vi "main.vi"() -> ()   [LabVIEW 2024]
uses:
  controls/#typedef_octave.ctl
  controls/#typedef_program_data.ctl
  <vilib>/sound2/lvsound2.llb/Sound Output Task ID.ctl
  controls/#typedef_audio_settings.ctl
  <vilib>/sound2/lvsound2.llb/Sound Data Format.ctl
  controls/#typedef_monitoring.ctl
  controls/#typedef_wave_settings.ctl
  controls/#typedef_wave_types.ctl
  controls/#typedef_ProgramStates.ctl
  <vilib>/sound2/lvsound2.llb/Sampling Mode.ctl
  controls/#typedef_action_timer.ctl
  <vilib>/Analysis/3filter.llb/Filter Passband Type.ctl
  <extravilib>/ChannelInstances/Tag-bool/Write With Abort.vi
  <extravilib>/ChannelInstances/Tag-bool/Read With Abort.vi
  <extravilib>/ChannelInstances/Tag-bool/Instantiate.vi
  <vilib>/Utility/file.llb/Read Delimited Spreadsheet (DBL).vi
  <vilib>/Analysis/3filter.llb/Butterworth Filter (DBL).vi
  <vilib>/sound2/lvsound2.llb/Sound Output Write (DBL Single).vi
  <vilib>/Analysis/3filter.llb/Bessel Filter (DBL).vi
  <extravilib>/ChannelInstances/Tag-bool/EndpointRead.vi
  <extravilib>/ChannelInstances/Tag-bool/Endpoint.vi
  <vilib>/Utility/file.llb/Write Delimited Spreadsheet (DBL).vi
  <vilib>/Analysis/NI_AALPro.lvlib
  <extravilib>/ChannelInstances/Tag-bool.lvlib
  <vilib>/Analysis/NI_AALBase.lvlib
panel:
  out "error out 2":errorcluster
  in  "error in (no error) 2":errorcluster
  out "String":string
  out "NAME":string
  in  "Open":bool
  in  "Save":bool
  in  "ON/OFF":bool
  in  "Transpose  ch 2":i16(knob) caption="Octave" scale=-3.0..3.0
  in  "frequency ch2":i32(knob) caption="Transpose" scale=0.0..12.0
  in  "Wave type 2":u16(knob) caption="Wave type" scale=0.0..3.0
  in  "Blend":dbl(knob) scale=0.0..1.0
  in  "Transpose ch 1":i16(knob) caption="Octave" scale=-3.0..3.0
  in  "Wave type":u16(knob) scale=0.0..3.0
  in  "Distortion":dbl(knob)=1.0 scale=0.0..1.0
  in  "LOW freq":dbl(knob) scale=1.0..11024.0 scale format="%#_6p"
  in  "HI freq":dbl(knob)=11025.0 scale=1.0..11025.0 scale format="%#_6p"
  in  "Program Data":T1={"task ID"=0, "Data"=[], "Frequecies"=[], "Audio Settings"={"device ID"=0, "Buffer Size"=64.0, "sound format"={"sample rate (S/s)"=22050.0, "number of channels"=2, "bits per sample"=16}, "Number of samples"=0}, "Monitoring"={"Pressed Key Nr"=0, "Played Freqency"=0.0, "Max Amplitude"=0.0, "Current Amplitude"=0.0, "Played Freqency 2"=0.0, "Played Freqency drone"=0.0}, "Wave settings"={"HI freq"=0.0, "LOW freq"=0.0, "wave type"=enum."Sine", "Distortion level"=0.0, "MIX volume"=0.0, "wave type 2"=enum."Sine", "wave type drone"=enum."Sine", "DRONE volume 2"=0.0}, "data"=[]} {"task ID" format="%.0x"}
  out "Waveform Graph":waveform(dbl)(graph)
  in  "Volume":dbl(knob)=0.279 caption="Master volume" scale=0.0..1.0
  in  "Attack":dbl(knob)=5.930889758440234 scale=0.0..10.0
  in  "Decay":dbl(knob)=5.530816944711532 scale=0.0..10.0
  in  "Octave 2":T8
  in  "Octave":T8
  out "error out":errorcluster
  in  "error in (no error)":errorcluster
  # "Channel 1"
  # "Channel 2"
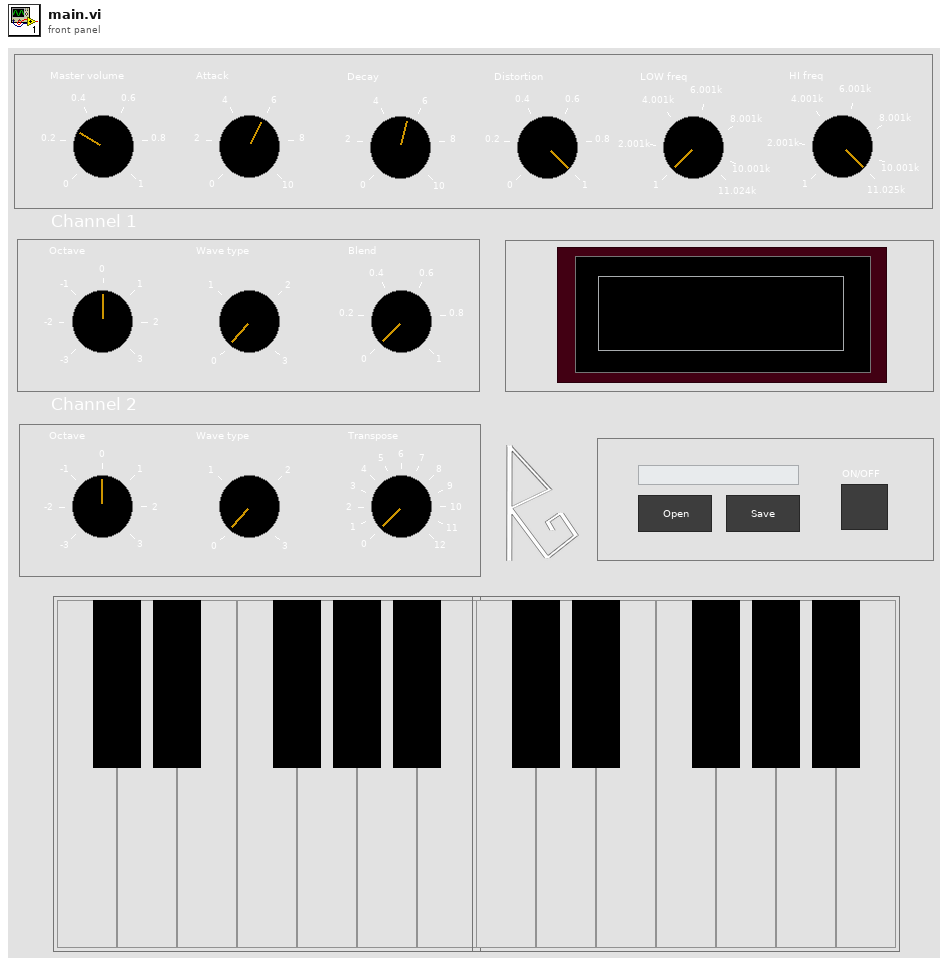
[diagram p1: front panel]
types:
  T1 = typedef "#typedef_program_data.ctl" = cluster{"task ID":T2, "Data":dbl[], "Frequecies":dbl[], "Audio Settings":T3, "Monitoring":T5, "Wave settings":T6, "data":waveform(dbl)[]}
  T2 = typedef "Sound Output Task ID.ctl" = u32
  T3 = typedef "#typedef_audio_settings.ctl" = cluster{"device ID":u32, "Buffer Size":dbl, "sound format":T4, "Number of samples":i32}
  T4 = typedef "Sound Data Format.ctl" = cluster{"sample rate (S/s)":dbl, "number of channels":i32, "bits per sample":i32}
  T5 = typedef "#typedef_monitoring.ctl" = cluster{"Pressed Key Nr":i32, "Played Freqency":dbl, "Max Amplitude":dbl, "Current Amplitude":dbl, "Played Freqency 2":dbl, "Played Freqency drone":dbl}
  T6 = typedef "#typedef_wave_settings.ctl" = cluster{"HI freq":dbl, "LOW freq":dbl, "wave type":T7, "Distortion level":dbl, "MIX volume":dbl, "wave type 2":T7, "wave type drone":T7, "DRONE volume 2":dbl}
  T7 = typedef "#typedef_wave_types.ctl" = enum16{"Sine", "Square", "Sawtooth", "Triangle"}
  T8 = typedef "#typedef_octave.ctl" = cluster{"C":bool, "D":bool, "E":bool, "F":bool, "G":bool, "C#":bool, "D#":bool, "A":bool, "G#":bool, "B":bool, "F#":bool, "Bb":bool}
  T9 = typedef "#typedef_ProgramStates.ctl" = enum16{"Application Error", "Settings", "Init", "logo", "Idle", "CheckNote", "Attack", "PlayNote", "Decay", "Release", "Exiting"}
  T10 = typedef "Tag-bool.lvlib/))Channel.ctl" = refnum<queue>
  T11 = typedef "#typedef_action_timer.ctl" = enum16{"reset", "timeElapsed"}
  T12 = typedef "NI_AALBase.lvlib/Filter Passband Type.ctl" = enum32{"Lowpass", "Highpass", "Bandpass", "Bandstop"}
  T13 = typedef "Sampling Mode.ctl" = i32
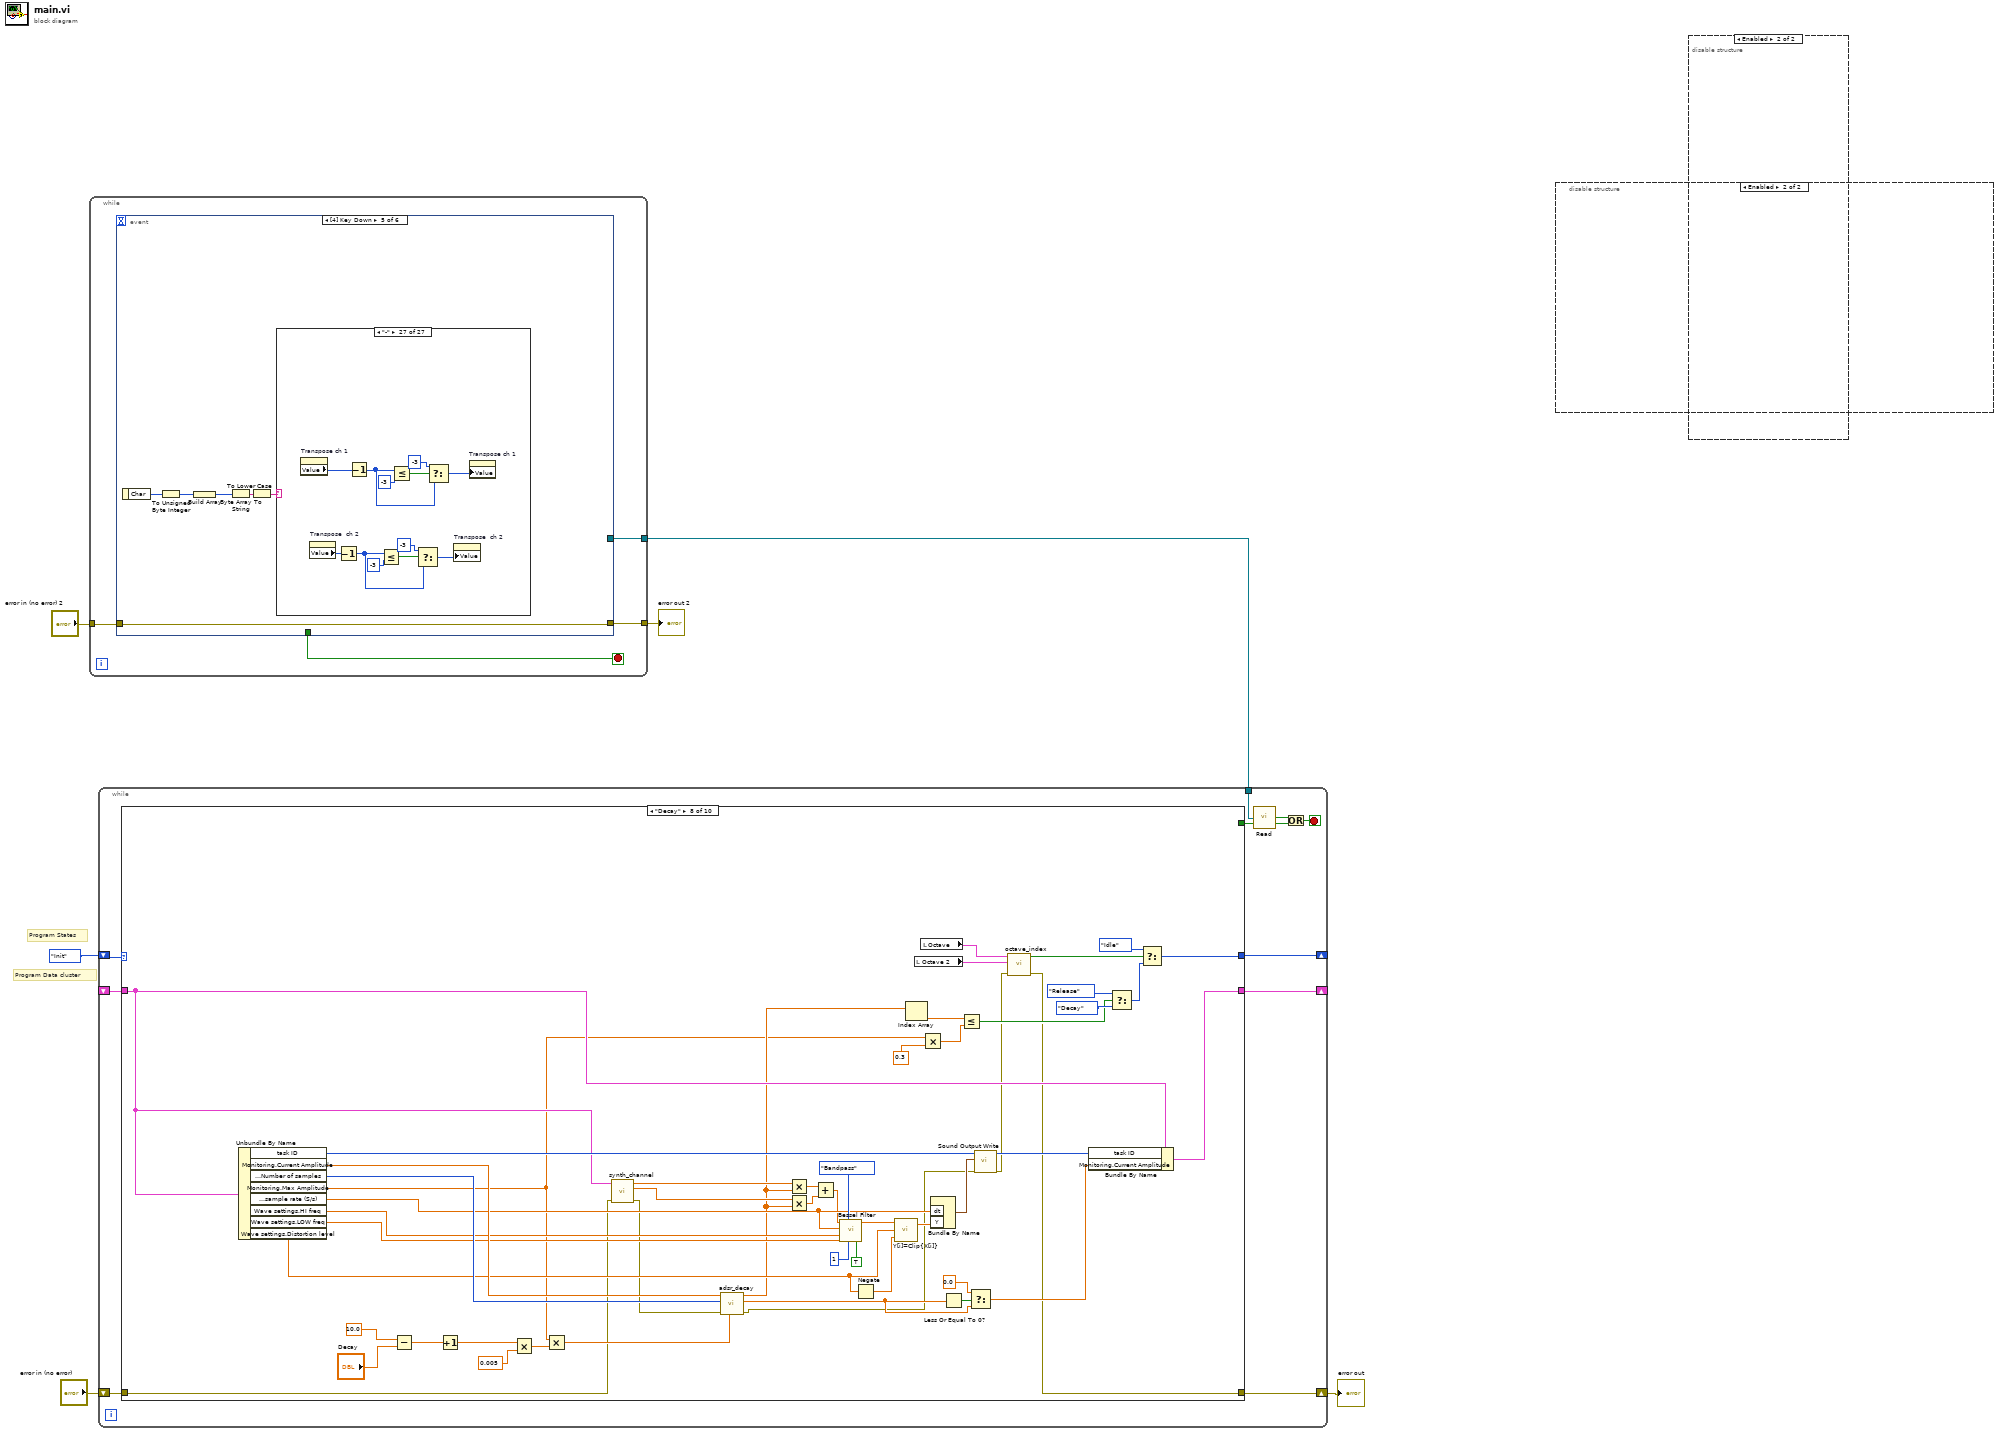
[diagram p0: block diagram]
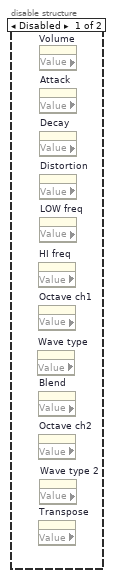
[diagram p2: hidden frame]
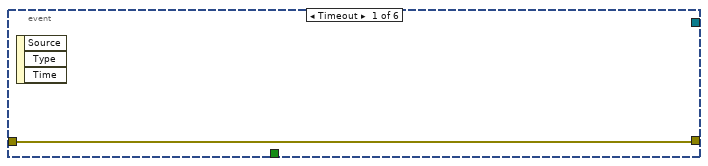
[diagram p3: hidden frame]
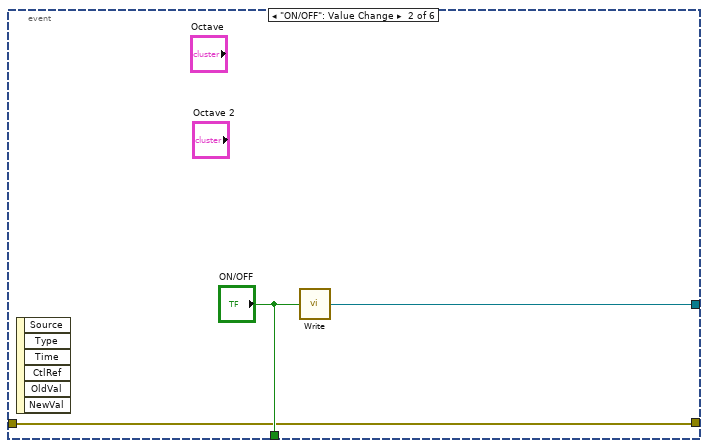
[diagram p4: hidden frame]
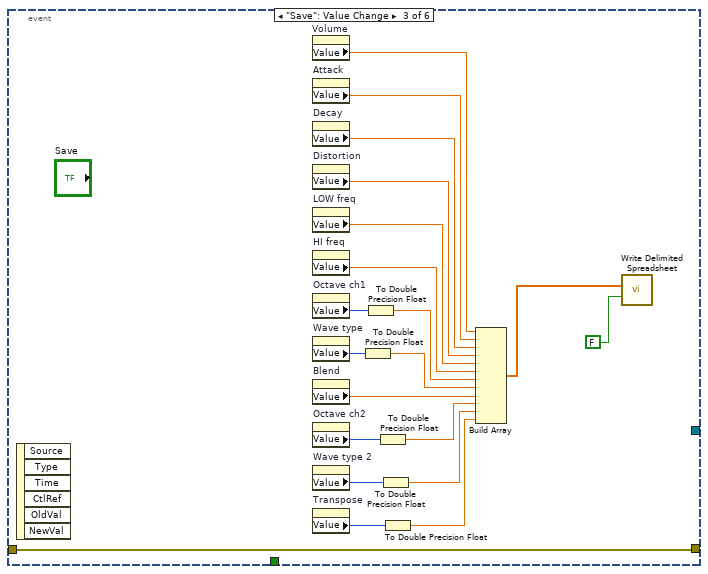
[diagram p5: hidden frame]
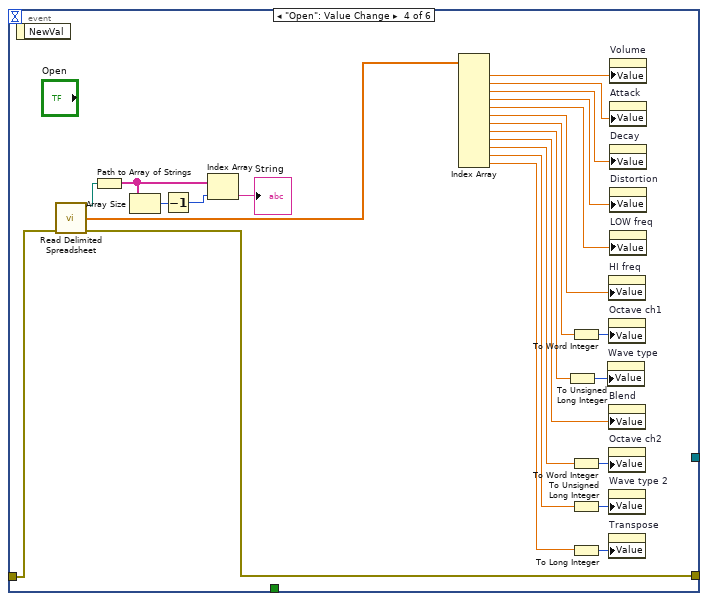
[diagram p6: hidden frame]
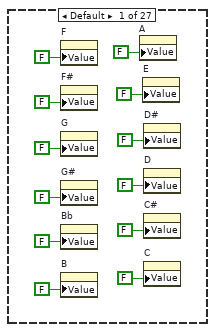
[diagram p7: hidden frame]
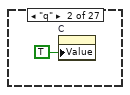
[diagram p8: hidden frame]
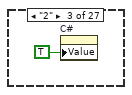
[diagram p9: hidden frame]
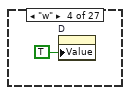
[diagram p10: hidden frame]
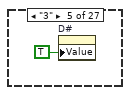
[diagram p11: hidden frame]
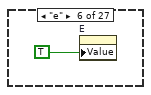
[diagram p12: hidden frame]
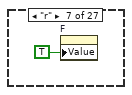
[diagram p13: hidden frame]
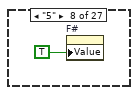
[diagram p14: hidden frame]
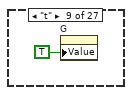
[diagram p15: hidden frame]
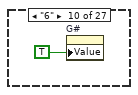
[diagram p16: hidden frame]
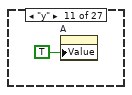
[diagram p17: hidden frame]
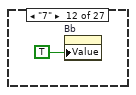
[diagram p18: hidden frame]
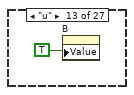
[diagram p19: hidden frame]
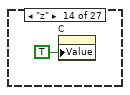
[diagram p20: hidden frame]
diagram:
  # "Program Data cluster"
  # "Program States"
  n1 = while {
    tunnel: [w9] -> w3
    tunnel: "error in (no error) 2" -> [w8]
    tunnel: [w7] -> w1
    stop <- w10 stop-if-true
    n2 = event shown="[4] Key Down" {
      selector: _ -> [_ _ _ _ _ _]
      dyn-events: _ -> [_ _ _ _ _ _]
      timeout: _ -> [_ _ _ _ _ _]
      tunnel: [_ "ON/OFF" _ _ _ _] -> w10
      tunnel: [_ w13 _ _ _ _] -> w9
      tunnel: w8 -> [w11 w12 w15 w54 w60 w126]
      tunnel: [w11 w12 w15 w53 w60 w126] -> w7
      event Timeout {
        n3 = event-data() -> ()  [unwired: 1 in, 3 out]
      }
      event "ON/OFF": Value Change {
        n4 = event-data() -> ()  [unwired: 1 in, 6 out]
        n5 = call <extravilib>:"Write.vi"("element"="ON/OFF") -> ("channel"=w13:T10)  [unwired: 1 out]
      }
      event "Save": Value Change {
        n6 = event-data() -> ()  [unwired: 1 in, 6 out]
        n7 = property on="Volume" class="Knob (strict)"() -> ("Value"=w32:dbl)  [unwired: 2 in, 2 out]
        n8 = property on="Attack" class="Knob (strict)"() -> ("Value"=w31:dbl)  [unwired: 2 in, 2 out]
        n9 = property on="Decay" class="Knob (strict)"() -> ("Value"=w30:dbl)  [unwired: 2 in, 2 out]
        n10 = property on="Distortion" class="Knob (strict)"() -> ("Value"=w29:dbl)  [unwired: 2 in, 2 out]
        n11 = property on="LOW freq" class="Knob (strict)"() -> ("Value"=w28:dbl)  [unwired: 2 in, 2 out]
        n12 = property on="HI freq" class="Knob (strict)"() -> ("Value"=w27:dbl)  [unwired: 2 in, 2 out]
        n13 = property on="Octave ch1" class="Knob (strict)"() -> ("Value"=w26:i16)  [unwired: 2 in, 2 out]
        n14 = property on="Wave type" class="Knob (strict)"() -> ("Value"=w17:u16)  [unwired: 2 in, 2 out]
        n15 = property on="Blend" class="Knob (strict)"() -> ("Value"=w25:dbl)  [unwired: 2 in, 2 out]
        n16 = property on="Octave ch2" class="Knob (strict)"() -> ("Value"=w24:i16)  [unwired: 2 in, 2 out]
        n17 = property on="Wave type 2" class="Knob (strict)"() -> ("Value"=w16:u16)  [unwired: 2 in, 2 out]
        n18 = property on="Transpose" class="Knob (strict)"() -> ("Value"=w23:i32)  [unwired: 2 in, 2 out]
        n19 = To Double Precision Float(number=w17) -> (double precision float=w19:dbl)
        n20 = To Double Precision Float(number=w26) -> (double precision float=w18:dbl)
        n21 = To Double Precision Float(number=w24) -> (double precision float=w20:dbl)
        n22 = To Double Precision Float(number=w16) -> (double precision float=w21:dbl)
        n23 = To Double Precision Float(number=w23) -> (double precision float=w22:dbl)
        n24 = Build Array(w32, w31, w30, w29, w28, w27, w18, w19, w25, w20, w21, w22) -> (w33:dbl[])
        n25 = call-poly <vilib>:"Write Delimited Spreadsheet.vi"("1D data"=w33, "append to file? (new file:F)"=FALSE) -> ()  [unwired: 12 in, 2 out]
      }
      event "Open": Value Change {
        n26 = event-data() -> ()  [unwired: 1 in, 1 out]
        n27 = call-poly <vilib>:"Read Delimited Spreadsheet.vi"("error in (no error)"=w54) -> ("new file path (Not A Path if cancelled)"=w59:path, "first row"=w36:dbl[], "error out"=w53:errorcluster)  [unwired: 9 in, 3 out]
        n28 = Path to Array of Strings(0:w59) -> (2:w57:string[])  [unwired: 1 out]
        n29 = Array Size(array=w57) -> (size(s)=w58:i32)
        n30 = Decrement(x=w58) -> (x-1=w56:i32)
        n31 = Index Array(array=w57, index=w56) -> (element=→"String":string)
        n32 = Index Array(array=w36) -> (element #1=w52:dbl, element #2=w46:dbl, element #3=w45:dbl, element #4=w44:dbl, element #5=w43:dbl, element #6=w42:dbl, element #7=w41:dbl, element #8=w40:dbl, element #9=w39:dbl, element #10=w38:dbl, element #11=w37:dbl, element #12=w35:dbl)  [unwired: 12 in]
        n33 = To Unsigned Long Integer(number=w40) -> (unsigned 32bit integer=w47:u32)
        n34 = To Word Integer(number=w41) -> (16bit integer=w51:i16)
        n35 = To Word Integer(number=w38) -> (16bit integer=w49:i16)
        n36 = To Unsigned Long Integer(number=w37) -> (unsigned 32bit integer=w48:u32)
        n37 = To Long Integer(number=w35) -> (32bit integer=w50:i32)
        n38 = property on="Wave type" class="Knob (strict)"("Value"=w47) -> ()  [unwired: 2 in, 2 out]
        n39 = property on="HI freq" class="Knob (strict)"("Value"=w42) -> ()  [unwired: 2 in, 2 out]
        n40 = property on="Octave ch1" class="Knob (strict)"("Value"=w51) -> ()  [unwired: 2 in, 2 out]
        n41 = property on="Blend" class="Knob (strict)"("Value"=w39) -> ()  [unwired: 2 in, 2 out]
        n42 = property on="Octave ch2" class="Knob (strict)"("Value"=w49) -> ()  [unwired: 2 in, 2 out]
        n43 = property on="Wave type 2" class="Knob (strict)"("Value"=w48) -> ()  [unwired: 2 in, 2 out]
        n44 = property on="Transpose" class="Knob (strict)"("Value"=w50) -> ()  [unwired: 2 in, 2 out]
        n45 = property on="Volume" class="Knob (strict)"("Value"=w52) -> ()  [unwired: 2 in, 2 out]
        n46 = property on="Attack" class="Knob (strict)"("Value"=w46) -> ()  [unwired: 2 in, 2 out]
        n47 = property on="Decay" class="Knob (strict)"("Value"=w45) -> ()  [unwired: 2 in, 2 out]
        n48 = property on="Distortion" class="Knob (strict)"("Value"=w44) -> ()  [unwired: 2 in, 2 out]
        n49 = property on="LOW freq" class="Knob (strict)"("Value"=w43) -> ()  [unwired: 2 in, 2 out]
      }
      event Key Down {
        n50 = event-data() -> ("Char"=w63:i16)  [unwired: 1 in]
        n51 = To Unsigned Byte Integer(number=w63) -> (unsigned 8bit integer=w65:u8)
        n52 = Build Array(w65) -> (w64:u8[])
        n53 = Byte Array To String(unsigned byte array=w64) -> (string=w62:string)
        n54 = To Lower Case(string=w62) -> (all lower case string=w61:string)
        n55 = case shown="\"-\"" w61 {
          frame Default {
            n56 = property on="F" class="Bool (strict)"("Value"=FALSE) -> ()  [unwired: 2 in, 2 out]
            n57 = property on="F#" class="Bool (strict)"("Value"=FALSE) -> ()  [unwired: 2 in, 2 out]
            n58 = property on="G" class="Bool (strict)"("Value"=FALSE) -> ()  [unwired: 2 in, 2 out]
            n59 = property on="G#" class="Bool (strict)"("Value"=FALSE) -> ()  [unwired: 2 in, 2 out]
            n60 = property on="Bb" class="Bool (strict)"("Value"=FALSE) -> ()  [unwired: 2 in, 2 out]
            n61 = property on="B" class="Bool (strict)"("Value"=FALSE) -> ()  [unwired: 2 in, 2 out]
            n62 = property on="A" class="Bool (strict)"("Value"=FALSE) -> ()  [unwired: 2 in, 2 out]
            n63 = property on="E" class="Bool (strict)"("Value"=FALSE) -> ()  [unwired: 2 in, 2 out]
            n64 = property on="D#" class="Bool (strict)"("Value"=FALSE) -> ()  [unwired: 2 in, 2 out]
            n65 = property on="D" class="Bool (strict)"("Value"=FALSE) -> ()  [unwired: 2 in, 2 out]
            n66 = property on="C#" class="Bool (strict)"("Value"=FALSE) -> ()  [unwired: 2 in, 2 out]
            n67 = property on="C" class="Bool (strict)"("Value"=FALSE) -> ()  [unwired: 2 in, 2 out]
          }
          frame "q" {
            n68 = property on="C" class="Bool (strict)"("Value"=TRUE) -> ()  [unwired: 2 in, 2 out]
          }
          frame "2" {
            n69 = property on="C#" class="Bool (strict)"("Value"=TRUE) -> ()  [unwired: 2 in, 2 out]
          }
          frame "w" {
            n70 = property on="D" class="Bool (strict)"("Value"=TRUE) -> ()  [unwired: 2 in, 2 out]
          }
          frame "3" {
            n71 = property on="D#" class="Bool (strict)"("Value"=TRUE) -> ()  [unwired: 2 in, 2 out]
          }
          frame "e" {
            n72 = property on="E" class="Bool (strict)"("Value"=TRUE) -> ()  [unwired: 2 in, 2 out]
          }
          frame "r" {
            n73 = property on="F" class="Bool (strict)"("Value"=TRUE) -> ()  [unwired: 2 in, 2 out]
          }
          frame "5" {
            n74 = property on="F#" class="Bool (strict)"("Value"=TRUE) -> ()  [unwired: 2 in, 2 out]
          }
          frame "t" {
            n75 = property on="G" class="Bool (strict)"("Value"=TRUE) -> ()  [unwired: 2 in, 2 out]
          }
          frame "6" {
            n76 = property on="G#" class="Bool (strict)"("Value"=TRUE) -> ()  [unwired: 2 in, 2 out]
          }
          frame "y" {
            n77 = property on="A" class="Bool (strict)"("Value"=TRUE) -> ()  [unwired: 2 in, 2 out]
          }
          frame "7" {
            n78 = property on="Bb" class="Bool (strict)"("Value"=TRUE) -> ()  [unwired: 2 in, 2 out]
          }
          frame "u" {
            n79 = property on="B" class="Bool (strict)"("Value"=TRUE) -> ()  [unwired: 2 in, 2 out]
          }
          frame "z" {
            n80 = property on="C" class="Bool (strict)"("Value"=TRUE) -> ()  [unwired: 2 in, 2 out]
          }
          frame "s" {
            n81 = property on="C#" class="Bool (strict)"("Value"=TRUE) -> ()  [unwired: 2 in, 2 out]
          }
          frame "x" {
            n82 = property on="D" class="Bool (strict)"("Value"=TRUE) -> ()  [unwired: 2 in, 2 out]
          }
          frame "d" {
            n83 = property on="D#" class="Bool (strict)"("Value"=TRUE) -> ()  [unwired: 2 in, 2 out]
          }
          frame "c" {
            n84 = property on="E" class="Bool (strict)"("Value"=TRUE) -> ()  [unwired: 2 in, 2 out]
          }
          frame "v" {
            n85 = property on="F" class="Bool (strict)"("Value"=TRUE) -> ()  [unwired: 2 in, 2 out]
          }
          frame "g" {
            n86 = property on="F#" class="Bool (strict)"("Value"=TRUE) -> ()  [unwired: 2 in, 2 out]
          }
          frame "b" {
            n87 = property on="G" class="Bool (strict)"("Value"=TRUE) -> ()  [unwired: 2 in, 2 out]
          }
          frame "h" {
            n88 = property on="G#" class="Bool (strict)"("Value"=TRUE) -> ()  [unwired: 2 in, 2 out]
          }
          frame "n" {
            n89 = property on="A" class="Bool (strict)"("Value"=TRUE) -> ()  [unwired: 2 in, 2 out]
          }
          frame "j" {
            n90 = property on="Bb" class="Bool (strict)"("Value"=TRUE) -> ()  [unwired: 2 in, 2 out]
          }
          frame "m" {
            n91 = property on="B" class="Bool (strict)"("Value"=TRUE) -> ()  [unwired: 2 in, 2 out]
          }
          frame "=" {
            n92 = property on="Transpose  ch 2" class="Knob (strict)"() -> ("Value"=w102:i16)  [unwired: 2 in, 2 out]
            n93 = property on="Transpose ch 1" class="Knob (strict)"() -> ("Value"=w113:i16)  [unwired: 2 in, 2 out]
            n94 = Increment(x=w102) -> (x+1=w104:i16)
            n95 = Increment(x=w113) -> (x+1=w109:i16)
            n96 = Greater Or Equal?(x=w104, y=i16 3) -> (x >= y?=w107:bool)
            n97 = Greater Or Equal?(x=w109, y=i16 3) -> (x >= y?=w112:bool)
            n98 = Select(t=i16 3 ("y"), s=w107, f=w104) -> (s? t:f=w103:i16)
            n99 = Select(t=i16 3 ("y"), s=w112, f=w109) -> (s? t:f=w108:i16)
            n100 = property on="Transpose  ch 2" class="Knob (strict)"("Value"=w103) -> ()  [unwired: 2 in, 2 out]
            n101 = property on="Transpose ch 1" class="Knob (strict)"("Value"=w108) -> ()  [unwired: 2 in, 2 out]
          }
          frame "-" {
            n102 = property on="Transpose ch 1" class="Knob (strict)"() -> ("Value"=w125:i16)  [unwired: 2 in, 2 out]
            n103 = property on="Transpose  ch 2" class="Knob (strict)"() -> ("Value"=w116:i16)  [unwired: 2 in, 2 out]
            n104 = Decrement(x=w116) -> (x-1=w117:i16)
            n105 = Decrement(x=w125) -> (x-1=w120:i16)
            n106 = Less Or Equal?(x=w117, y=i16 -3) -> (x <= y?=w119:bool)
            n107 = Less Or Equal?(x=w120, y=i16 -3) -> (x <= y?=w124:bool)
            n108 = Select(t=i16 -3 ("y"), s=w119, f=w117) -> (s? t:f=w115:i16)
            n109 = Select(t=i16 -3 ("y"), s=w124, f=w120) -> (s? t:f=w121:i16)
            n110 = property on="Transpose  ch 2" class="Knob (strict)"("Value"=w115) -> ()  [unwired: 2 in, 2 out]
            n111 = property on="Transpose ch 1" class="Knob (strict)"("Value"=w121) -> ()  [unwired: 2 in, 2 out]
          }
        }
      }
      event Key Up {
        n112 = event-data() -> ()  [unwired: 1 in, 7 out]
        n113 = property on="D" class="Bool (strict)"("Value"=FALSE) -> ()  [unwired: 2 in, 2 out]
        n114 = property on="D#" class="Bool (strict)"("Value"=FALSE) -> ()  [unwired: 2 in, 2 out]
        n115 = property on="C#" class="Bool (strict)"("Value"=FALSE) -> ()  [unwired: 2 in, 2 out]
        n116 = property on="C" class="Bool (strict)"("Value"=FALSE) -> ()  [unwired: 2 in, 2 out]
        n117 = property on="G" class="Bool (strict)"("Value"=FALSE) -> ()  [unwired: 2 in, 2 out]
        n118 = property on="F" class="Bool (strict)"("Value"=FALSE) -> ()  [unwired: 2 in, 2 out]
        n119 = property on="F#" class="Bool (strict)"("Value"=FALSE) -> ()  [unwired: 2 in, 2 out]
        n120 = property on="E" class="Bool (strict)"("Value"=FALSE) -> ()  [unwired: 2 in, 2 out]
        n121 = property on="G#" class="Bool (strict)"("Value"=FALSE) -> ()  [unwired: 2 in, 2 out]
        n122 = property on="Bb" class="Bool (strict)"("Value"=FALSE) -> ()  [unwired: 2 in, 2 out]
        n123 = property on="B" class="Bool (strict)"("Value"=FALSE) -> ()  [unwired: 2 in, 2 out]
        n124 = property on="A" class="Bool (strict)"("Value"=FALSE) -> ()  [unwired: 2 in, 2 out]
        n125 = property on="B" class="Bool (strict)"("Value"=FALSE) -> ()  [unwired: 2 in, 2 out]
        n126 = property on="Bb" class="Bool (strict)"("Value"=FALSE) -> ()  [unwired: 2 in, 2 out]
        n127 = property on="A" class="Bool (strict)"("Value"=FALSE) -> ()  [unwired: 2 in, 2 out]
        n128 = property on="F#" class="Bool (strict)"("Value"=FALSE) -> ()  [unwired: 2 in, 2 out]
        n129 = property on="F" class="Bool (strict)"("Value"=FALSE) -> ()  [unwired: 2 in, 2 out]
        n130 = property on="G" class="Bool (strict)"("Value"=FALSE) -> ()  [unwired: 2 in, 2 out]
        n131 = property on="G#" class="Bool (strict)"("Value"=FALSE) -> ()  [unwired: 2 in, 2 out]
        n132 = property on="E" class="Bool (strict)"("Value"=FALSE) -> ()  [unwired: 2 in, 2 out]
        n133 = property on="D#" class="Bool (strict)"("Value"=FALSE) -> ()  [unwired: 2 in, 2 out]
        n134 = property on="D" class="Bool (strict)"("Value"=FALSE) -> ()  [unwired: 2 in, 2 out]
        n135 = property on="C#" class="Bool (strict)"("Value"=FALSE) -> ()  [unwired: 2 in, 2 out]
        n136 = property on="C" class="Bool (strict)"("Value"=FALSE) -> ()  [unwired: 2 in, 2 out]
      }
    }
  }
  "error out 2" <- w1
  n137 = while {
    shift-right: [w158] -> _
    shift-left: #typedef_ProgramStates."Init" ("ProgramStates") -> [w160]
    shift-right: [w151] -> _
    shift-left: _ -> [w159]
    shift-right: [w155] -> w4
    shift-left: "error in (no error)" -> [w156]
    tunnel: w3 -> [w153]
    stop <- w154 stop-if-true
    n138 = case shown="\"Decay\"" w160 {
      selector: w160 -> [w167 _ _ _ _ _ _ _ _ _]
      tunnel: w159 -> [w168 w171 _ w227 w237 w268 w319 w357 w407 w439]
      tunnel: [w168 w171 w211 w227 w260 w308 w339 w391 w438 w439] -> w151
      tunnel: [#typedef_ProgramStates."Exiting" ("ProgramStates") #typedef_ProgramStates."Idle" ("ProgramStates") #typedef_ProgramStates."logo" ("ProgramStates") w223 w234 w297 w332 w388 w435 #typedef_ProgramStates."Application Error" ("ProgramStates")] -> w158
      tunnel: [w163 _ _ _ _ _ _ _ _ TRUE] -> w157
      tunnel: [w161 w170 w184 w220 w238 w264 w310 w343 w393 w440] -> w155
      tunnel: w156 -> [w161 w170 w210 w221 w239 w266 w314 w345 w397 w441]
      frame "Application Error", Default {
        n139 = Format Into String(w167) -> (resulting string=w166:string)  [unwired: 3 in, 1 out]
        n140 = Two Button Dialog(message=w166, 1:"Terminate with exiting" ("F button name (\"Cancel\")"), 2:"Terminate" ("T button name (\"OK\")")) -> (T button?=w163:bool)
      }
      frame "Settings" {
      }
      frame "Init" {
        w214 = T13 1 items=["Finite Samples", "Continuous Samples"] ("sample mode")
        n141 = Bundle By Name(cluster="Program Data", "Audio Settings.Buffer Size"=64.0) -> (w209:T1)
        n142 = Unbundle By Name(w209) -> ("Audio Settings.sound format.sample rate (S/s)"=w219:dbl, "Audio Settings.Buffer Size"=w218:dbl, "Audio Settings.device ID"=w217:u32, "Audio Settings.sound format"=w216:T4, "Audio Settings.sound format.sample rate (S/s)"=w204:dbl)
        n143 = Divide(x=w204, y=2.0) -> (x/y=w202:dbl)
        n144 = Decrement(x=w202) -> (x-1=w201:dbl)
        n145 = property on="HI freq" class="Knob (strict)"("Scale.Maximum"=w202) -> ()  [unwired: 2 in, 2 out]
        n146 = property on="LOW freq" class="Knob (strict)"("Scale.Maximum"=w201) -> ()  [unwired: 2 in, 2 out]
        n147 = Divide(x=w219, y=w218) -> (x/y=w215:dbl)
        n148 = To Long Integer(number=w215) -> (32bit integer=w212:i32)
        n149 = call <vilib>:"Sound Output Configure.vi"("number of samples/ch"=w212, "sample mode"=w214, "error in (no error)"=w210, "sound format"=w216, "device ID"=w217) -> ("error out"=w186:errorcluster, "task ID"=w213:T2)  [unwired: 5 in]
        n150 = call <vilib>:"Application Directory.vi"() -> ("Application Directory"=w189:path)
        n151 = Build Path(base path=w189, name or relative path=path "synth/Files/presets/electro 3") -> (appended path=w187:path)
        n152 = call-poly <vilib>:"Read Delimited Spreadsheet.vi"("file path (dialog if empty)"=w187, "error in (no error)"=w186) -> ("first row"=w194:dbl[], "error out"=w185:errorcluster)  [unwired: 8 in, 4 out]
        n153 = property on="Volume" class="Knob (strict)"() -> ("Value"=w206:dbl)  [unwired: 2 in, 2 out]
        n154 = property on="Distortion" class="Knob (strict)"() -> ("Value"=w200:dbl)  [unwired: 2 in, 2 out]
        n155 = Index Array(array=w194) -> (element #1=w195:dbl, element #2=w182:dbl, element #3=w181:dbl, element #4=w180:dbl, element #5=w179:dbl, element #6=w178:dbl, element #7=w177:dbl, element #8=w176:dbl, element #9=w175:dbl, element #10=w174:dbl, element #11=w173:dbl, element #12=w172:dbl)  [unwired: 12 in]
        n156 = Bundle By Name(cluster="Program Data", "Frequecies"=dbl[] [261.626, 277.183, 293.665, 311.127, 329.628, 349.228, 369.994, 391.995, 415.305, 440.0, 466.164, 493.883, 523.2511, 554.3653, 587.3295, 622.254, 659.2551, 698.4565, 739.9888, 783.9909, 830.6094, 880.0, 932.3275, 987.7666, 1046.502, 1108.731, 1174.659, 1244.508, 1328.51, 1396.913, 1479.978, 1567.982, 1661.219, 1760.0, 1864.655, 1975.533, 2093.005], "Audio Settings.Number of samples"=w212, "task ID"=w213, "Monitoring.Current Amplitude"=0.0 ("Current Amplitude"), "Monitoring.Max Amplitude"=w206, "Wave settings.Distortion level"=w200) -> (w211:T1)
        n157 = To Unsigned Long Integer(number=w176) -> (unsigned 32bit integer=w183:u32)
        n158 = To Word Integer(number=w177) -> (16bit integer=w193:i16)
        n159 = To Word Integer(number=w174) -> (16bit integer=w191:i16)
        n160 = To Unsigned Long Integer(number=w173) -> (unsigned 32bit integer=w190:u32)
        n161 = To Long Integer(number=w172) -> (32bit integer=w192:i32)
        n162 = property on="Wave type" class="Knob (strict)"("Value"=w183) -> ()  [unwired: 2 in, 2 out]
        n163 = property on="HI freq" class="Knob (strict)"("Value"=w178) -> ()  [unwired: 2 in, 2 out]
        n164 = property on="Octave ch1" class="Knob (strict)"("Value"=w193) -> ()  [unwired: 2 in, 2 out]
        n165 = property on="Blend" class="Knob (strict)"("Value"=w175) -> ()  [unwired: 2 in, 2 out]
        n166 = property on="Octave ch2" class="Knob (strict)"("Value"=w191) -> ()  [unwired: 2 in, 2 out]
        n167 = property on="Wave type 2" class="Knob (strict)"("Value"=w190) -> ()  [unwired: 2 in, 2 out]
        n168 = property on="Transpose" class="Knob (strict)"("Value"=w192) -> ()  [unwired: 2 in, 2 out]
        n169 = property on="Volume" class="Knob (strict)"("Value"=w195) -> ()  [unwired: 2 in, 2 out]
        n170 = property on="Attack" class="Knob (strict)"("Value"=w182) -> ()  [unwired: 2 in, 2 out]
        n171 = property on="Decay" class="Knob (strict)"("Value"=w181) -> ()  [unwired: 2 in, 2 out]
        n172 = property on="Distortion" class="Knob (strict)"("Value"=w180) -> ()  [unwired: 2 in, 2 out]
        n173 = property on="LOW freq" class="Knob (strict)"("Value"=w179) -> ()  [unwired: 2 in, 2 out]
        n174 = property on="String" class="Str"("Value"="Select preset" ("String")) -> ()  [unwired: 2 in, 2 out]
        n175 = call "timer.vi"("error in (no error)"=w185, "action"=#typedef_action_timer."reset") -> ("error out"=w184:errorcluster)  [unwired: 6 in, 3 out]
      }
      frame "logo" {
        n176 = call "timer.vi"("error in (no error)"=w221, "action"=#typedef_action_timer."timeElapsed", "Time to elapse (s)"=1.0) -> ("error out"=w220:errorcluster, "timeElapsed?"=w226:bool)  [unwired: 5 in, 2 out]
        n177 = case shown="True" w226 {
          tunnel: [#typedef_ProgramStates."logo" ("ProgramStates") #typedef_ProgramStates."Idle" ("ProgramStates")] -> w223
          frame False {
            n178 = property on="Waveform Graph" class="WFGraph (strict)"("Plot.Visible?"=FALSE ("Plot.Visible")) -> ()  [unwired: 2 in, 2 out]
            n179 = property on="NAME" class="Str"("Visible"=TRUE) -> ()  [unwired: 2 in, 2 out]
          }
          frame True {
            n180 = property on="Waveform Graph" class="WFGraph (strict)"("Plot.Visible?"=TRUE ("Plot.Visible")) -> ()  [unwired: 2 in, 2 out]
            n181 = property on="NAME" class="Str"("Visible"=FALSE) -> ()  [unwired: 2 in, 2 out]
          }
        }
        "NAME" <- "Wavemix" ("String 2")
      }
      frame "Idle" {
        n182 = Unbundle By Name(w237) -> ("Frequecies"=w242:dbl[])
        n183 = local read "Octave 2"() -> (w241:T8)
        n184 = local read "Octave"() -> (w256:T8)
        n185 = call "octave_index.vi"("error in (no error)"=w239, "Octave 2"=w241, "Octave"=w256) -> ("error out"=w238:errorcluster, "max index(es)"=w240:i32, "Is key pressed?"=w257:bool)  [unwired: 5 in, 1 out]
        n186 = Add(x=w240, y="frequency ch2") -> (x+y=w244:i32)
        n187 = Index Array(array=w242, index=w240) -> (element=w255:dbl)
        n188 = Index Array(array=w242, index=w244) -> (element=w245:dbl)
        n189 = Scale By Power Of 2(n="Transpose ch 1", x=w255) -> (x*2^n=w254:dbl)
        n190 = Scale By Power Of 2(n="Transpose  ch 2", x=w245) -> (x*2^n=w243:dbl)
        n191 = Bundle By Name(cluster=w237, "Monitoring.Played Freqency 2"=w243, "Monitoring.Played Freqency"=w254, "Monitoring.Max Amplitude"="Volume", "Wave settings.HI freq"="HI freq", "Wave settings.LOW freq"="LOW freq", "Wave settings.Distortion level"="Distortion", "Wave settings.MIX volume"="Blend", "Wave settings.wave type"="Wave type", "Wave settings.wave type 2"="Wave type 2") -> (w260:T1)
        n192 = Select(t=#typedef_ProgramStates."Attack" ("ProgramStates"), s=w257, f=#typedef_ProgramStates."Idle") -> (s? t:f=w234:T9)
      }
      frame "Attack" {
        n193 = Unbundle By Name(w268) -> ("task ID"=w306:T2, "Monitoring.Max Amplitude"=w290:dbl, "Monitoring.Current Amplitude"=w295:dbl, "Audio Settings.Number of samples"=w294:i32, "Monitoring.Max Amplitude"=w285:dbl, "Audio Settings.sound format.sample rate (S/s)"=w283:dbl, "Wave settings.HI freq"=w282:dbl, "Wave settings.LOW freq"=w281:dbl, "Wave settings.Distortion level"=w275:dbl)
        n194 = Subtract(x=10.0, y="Attack") -> (x-y=w286:dbl)
        n195 = Increment(x=w286) -> (x+1=w274:dbl)
        n196 = call "synth_channel.vi"("error in (no error)"=w266, "Program Data"=w268) -> ("error out"=w263:errorcluster, "output wave 2"=w270:dbl[], "output wave"=w296:dbl[])  [unwired: 7 in]
        n197 = Multiply(x=w285, y=w274) -> (x*y=w292:dbl)
        n198 = Multiply(x=0.005 ("y"), y=w292) -> (x*y=w291:dbl)
        n199 = local read "Octave 2"() -> (w267:T8)
        n200 = local read "Octave"() -> (w301:T8)
        n201 = call "adsr_attack.vi"("Attack"=w291, "error in (no error)"=w263, "Number of samples"=w294, "Current Amplitude"=w295) -> ("error out"=w262:errorcluster, "Current amplitude"=w293:dbl, "Ramp Pattern"=w271:dbl[])  [unwired: 5 in]
        n202 = Multiply(x=w270, y=w271) -> (x*y=w269:dbl[])
        n203 = Multiply(x=w296, y=w271) -> (x*y=w284:dbl[])
        n204 = call "octave_index.vi"("error in (no error)"=w262, "Octave 2"=w267, "Octave"=w301) -> ("error out"=w265:errorcluster, "Is key pressed?"=w300:bool)  [unwired: 5 in, 2 out]
        n205 = Add(x=w284, y=w269) -> (x+y=w272:dbl[])
        n206 = Not(x=w300) -> (.not. x?=w298:bool)
        n207 = Less Or Equal?(x=w290, y=w295) -> (x <= y?=w299:bool)
        n208 = call-poly <vilib>:"Butterworth Filter.vi"("init/cont (init:F)"=TRUE, "order"=1, "filter type"=Filter_Passband_Type."Bandpass", "low cutoff freq: fl"=w281, "high cutoff freq: fh"=w282, "sampling freq: fs"=w283, "X"=w272) -> ("Filtered X"=w277:dbl[])  [unwired: 1 in, 1 out]
        n209 = Negate(x=w275) -> (-x=w276:dbl)
        n210 = call <vilib>:"Y[i]=Clip{X[i]}.vi"("lower limit"=w276, "upper limit"=w275, "Input Array"=w277) -> ("Clipped Array"=w273:dbl[])  [unwired: 1 out]
        n211 = Bundle By Name("Y"=w273, "dt"=w283) -> (w261:waveform(dbl))  [unwired: 1 in]
        "Waveform Graph" <- w261
        n212 = call-poly <vilib>:"Sound Output Write.vi"("error in (no error)"=w265, "data"=w261, "task ID"=w306) -> ("error out"=w264:errorcluster, "task ID out"=w307:T2)  [unwired: 7 in]
        n213 = Select(t=#typedef_ProgramStates."PlayNote" ("ProgramStates"), s=w299, f=#typedef_ProgramStates."Attack") -> (s? t:f=w302:T9)
        n214 = Bundle By Name(cluster=w268, "task ID"=w307, "Monitoring.Current Amplitude"=w293) -> (w308:T1)
        n215 = Select(t=#typedef_ProgramStates."Decay", s=w298, f=w302) -> (s? t:f=w297:T9)
      }
      frame "PlayNote" {
        n216 = Unbundle By Name(w319) -> ("task ID"=w337:T2, "Monitoring.Max Amplitude"=w317:dbl, "Audio Settings.sound format.sample rate (S/s)"=w329:dbl, "Wave settings.HI freq"=w326:dbl, "Wave settings.LOW freq"=w325:dbl, "Wave settings.Distortion level"=w321:dbl)  [unwired: 1 out]
        n217 = call "synth_channel.vi"("error in (no error)"=w314, "Program Data"=w319) -> ("error out"=w312:errorcluster, "output wave 2"=w316:dbl[], "output wave"=w331:dbl[])  [unwired: 7 in]
        n218 = Multiply(x=w316, y=w317) -> (x*y=w318:dbl[])
        n219 = Multiply(x=w331, y=w317) -> (x*y=w330:dbl[])
        n220 = Add(x=w330, y=w318) -> (x+y=w315:dbl[])
        n221 = call-poly <vilib>:"Butterworth Filter.vi"("init/cont (init:F)"=TRUE, "order"=1, "filter type"=Filter_Passband_Type."Bandpass", "low cutoff freq: fl"=w325, "high cutoff freq: fh"=w326, "sampling freq: fs"=w329, "X"=w315) -> ("Filtered X"=w323:dbl[])  [unwired: 1 in, 1 out]
        n222 = local read "Octave 2"() -> (w313:T8)
        n223 = Negate(x=w321) -> (-x=w322:dbl)
        n224 = local read "Octave"() -> (w333:T8)
        n225 = call <vilib>:"Y[i]=Clip{X[i]}.vi"("lower limit"=w322, "upper limit"=w321, "Input Array"=w323) -> ("Clipped Array"=w320:dbl[])  [unwired: 1 out]
        n226 = call "octave_index.vi"("error in (no error)"=w312, "Octave 2"=w313, "Octave"=w333) -> ("error out"=w311:errorcluster, "Is key pressed?"=w334:bool)  [unwired: 5 in, 2 out]
        n227 = Bundle By Name("Y"=w320, "dt"=w329) -> (w309:waveform(dbl))  [unwired: 1 in]
        n228 = call-poly <vilib>:"Sound Output Write.vi"("error in (no error)"=w311, "data"=w309, "task ID"=w337) -> ("error out"=w310:errorcluster, "task ID out"=w338:T2)  [unwired: 7 in]
        n229 = Select(t=#typedef_ProgramStates."PlayNote", s=w334, f=#typedef_ProgramStates."Decay" ("ProgramStates")) -> (s? t:f=w332:T9)
        n230 = Bundle By Name(cluster=w319, "task ID"=w338) -> (w339:T1)
      }
      frame "Decay" {
        n231 = Unbundle By Name(w357) -> ("task ID"=w389:T2, "Monitoring.Current Amplitude"=w379:dbl, "Audio Settings.Number of samples"=w380:i32, "Monitoring.Max Amplitude"=w347:dbl, "Audio Settings.sound format.sample rate (S/s)"=w365:dbl, "Wave settings.HI freq"=w370:dbl, "Wave settings.LOW freq"=w369:dbl, "Wave settings.Distortion level"=w362:dbl)
        n232 = Subtract(x=10.0, y="Decay") -> (x-y=w373:dbl)
        n233 = Increment(x=w373) -> (x+1=w376:dbl)
        n234 = Multiply(x=w376, y=0.005) -> (x*y=w377:dbl)
        n235 = Multiply(x=w347, y=w377) -> (x*y=w353:dbl)
        n236 = call "synth_channel.vi"("error in (no error)"=w345, "Program Data"=w357) -> ("error out"=w344:errorcluster, "output wave 2"=w361:dbl[], "output wave"=w381:dbl[])  [unwired: 7 in]
        n237 = call "adsr_decay.vi"("Decay"=w353, "error in (no error)"=w344, "Number of samples"=w380, "Current Amplitude"=w379) -> ("error out"=w341:errorcluster, "Current amplitude"=w354:dbl, "Ramp Pattern"=w352:dbl[])  [unwired: 5 in]
        n238 = Multiply(x=w381, y=w352) -> (x*y=w358:dbl[])
        n239 = Multiply(x=w361, y=w352) -> (x*y=w360:dbl[])
        n240 = Add(x=w358, y=w360) -> (x+y=w359:dbl[])
        n241 = call-poly <vilib>:"Bessel Filter.vi"("init/cont (init:F)"=TRUE, "order"=1, "filter type"=Filter_Passband_Type."Bandpass", "low cutoff freq: fl"=w369, "high cutoff freq: fh"=w370, "sampling freq: fs"=w365, "X"=w359) -> ("Filtered X"=w364:dbl[])  [unwired: 1 in, 1 out]
        n242 = Negate(x=w362) -> (-x=w363:dbl)
        n243 = call <vilib>:"Y[i]=Clip{X[i]}.vi"("lower limit"=w363, "upper limit"=w362, "Input Array"=w364) -> ("Clipped Array"=w355:dbl[])  [unwired: 1 out]
        n244 = Index Array(array=w352) -> (element=w351:dbl)  [unwired: 1 in]
        n245 = local read "Octave 2"() -> (w346:T8)
        n246 = local read "Octave"() -> (w382:T8)
        n247 = Multiply(x=w347, y=0.3) -> (x*y=w349:dbl)
        n248 = Bundle By Name("dt"=w365, "Y"=w355) -> (w342:waveform(dbl))  [unwired: 1 in]
        n249 = Less Or Equal To 0?(x=w354) -> (x <= 0?=w372:bool)
        n250 = Less Or Equal?(x=w351, y=w349) -> (x <= y?=w350:bool)
        n251 = Select(t=0.0, s=w372, f=w354) -> (s? t:f=w356:dbl)
        n252 = call-poly <vilib>:"Sound Output Write.vi"("error in (no error)"=w341, "data"=w342, "task ID"=w389) -> ("error out"=w340:errorcluster, "task ID out"=w390:T2)  [unwired: 7 in]
        n253 = call "octave_index.vi"("error in (no error)"=w340, "Octave 2"=w346, "Octave"=w382) -> ("error out"=w343:errorcluster, "Is key pressed?"=w387:bool)  [unwired: 5 in, 2 out]
        n254 = Bundle By Name(cluster=w357, "task ID"=w390, "Monitoring.Current Amplitude"=w356) -> (w391:T1)
        n255 = Select(t=#typedef_ProgramStates."Release" ("ProgramStates"), s=w350, f=#typedef_ProgramStates."Decay") -> (s? t:f=w383:T9)
        n256 = Select(t=#typedef_ProgramStates."Idle", s=w387, f=w383) -> (s? t:f=w388:T9)
      }
      frame "Release" {
        n257 = Unbundle By Name(w407) -> ("task ID"=w436:T2, "Monitoring.Current Amplitude"=w426:dbl, "Audio Settings.Number of samples"=w427:i32, "Monitoring.Max Amplitude"=w423:dbl, "Audio Settings.sound format.sample rate (S/s)"=w415:dbl, "Wave settings.HI freq"=w420:dbl, "Wave settings.LOW freq"=w419:dbl, "Wave settings.Distortion level"=w412:dbl)
        n258 = Multiply(x=1.0, y=0.005) -> (x*y=w424:dbl)
        n259 = Multiply(x=w423, y=w424) -> (x*y=w403:dbl)
        n260 = call "synth_channel.vi"("error in (no error)"=w397, "Program Data"=w407) -> ("error out"=w396:errorcluster, "output wave 2"=w411:dbl[], "output wave"=w428:dbl[])  [unwired: 7 in]
        n261 = call "adsr_decay.vi"("Decay"=w403, "error in (no error)"=w396, "Number of samples"=w427, "Current Amplitude"=w426) -> ("error out"=w395:errorcluster, "Current amplitude"=w404:dbl, "Ramp Pattern"=w402:dbl[])  [unwired: 5 in]
        n262 = Multiply(x=w428, y=w402) -> (x*y=w408:dbl[])
        n263 = Multiply(x=w411, y=w402) -> (x*y=w410:dbl[])
        n264 = Add(x=w408, y=w410) -> (x+y=w409:dbl[])
        n265 = call-poly <vilib>:"Bessel Filter.vi"("init/cont (init:F)"=TRUE, "order"=1, "filter type"=Filter_Passband_Type."Bandpass", "low cutoff freq: fl"=w419, "high cutoff freq: fh"=w420, "sampling freq: fs"=w415, "X"=w409) -> ("Filtered X"=w414:dbl[])  [unwired: 1 in, 1 out]
        n266 = Negate(x=w412) -> (-x=w413:dbl)
        n267 = call <vilib>:"Y[i]=Clip{X[i]}.vi"("lower limit"=w413, "upper limit"=w412, "Input Array"=w414) -> ("Clipped Array"=w405:dbl[])  [unwired: 1 out]
        n268 = Index Array(array=w402) -> (element=w400:dbl)  [unwired: 1 in]
        n269 = Bundle By Name("dt"=w415, "Y"=w405) -> (w392:waveform(dbl))  [unwired: 1 in]
        n270 = Less Or Equal To 0?(x=w400) -> (x <= 0?=w401:bool)
        n271 = local read "Octave 2"() -> (w398:T8)
        n272 = local read "Octave"() -> (w429:T8)
        n273 = call-poly <vilib>:"Sound Output Write.vi"("error in (no error)"=w395, "data"=w392, "task ID"=w436) -> ("error out"=w394:errorcluster, "task ID out"=w437:T2)  [unwired: 7 in]
        n274 = Less Or Equal To 0?(x=w404) -> (x <= 0?=w422:bool)
        n275 = Select(t=0.0, s=w422, f=w404) -> (s? t:f=w406:dbl)
        n276 = call "octave_index.vi"("error in (no error)"=w394, "Octave 2"=w398, "Octave"=w429) -> ("error out"=w393:errorcluster, "Is key pressed?"=w434:bool)  [unwired: 5 in, 2 out]
        n277 = Bundle By Name(cluster=w407, "task ID"=w437, "Monitoring.Current Amplitude"=w406) -> (w438:T1)
        n278 = Select(t=#typedef_ProgramStates."Idle" ("ProgramStates"), s=w401, f=#typedef_ProgramStates."Release") -> (s? t:f=w430:T9)
        n279 = Select(t=#typedef_ProgramStates."Idle", s=w434, f=w430) -> (s? t:f=w435:T9)
      }
      frame "Exiting" {
        n280 = Unbundle By Name(w439) -> ("task ID"=w442:T2)
        n281 = call <vilib>:"Sound Output Clear.vi"("error in (no error)"=w441, "task ID"=w442) -> ("error out"=w440:errorcluster)  [unwired: 9 in]
      }
    }
    n282 = call <extravilib>:"Read.vi"("channel"=w153) -> ("element"=w152:bool)  [unwired: 1 in, 1 out]
    n283 = Or(x=w152, y=w157) -> (x .or. y?=w154:bool)
  }
  "error out" <- w4
  n284 = disable-structure shown="Enabled" {
    frame Disabled {
      n285 = property on="F" class="Bool (strict)"("Value"=FALSE) -> ()  [unwired: 2 in, 2 out]
      n286 = property on="F#" class="Bool (strict)"("Value"=FALSE) -> ()  [unwired: 2 in, 2 out]
      n287 = property on="G" class="Bool (strict)"("Value"=FALSE) -> ()  [unwired: 2 in, 2 out]
      n288 = property on="G#" class="Bool (strict)"("Value"=FALSE) -> ()  [unwired: 2 in, 2 out]
      n289 = property on="Bb" class="Bool (strict)"("Value"=FALSE) -> ()  [unwired: 2 in, 2 out]
      n290 = property on="B" class="Bool (strict)"("Value"=FALSE) -> ()  [unwired: 2 in, 2 out]
      n291 = property on="A" class="Bool (strict)"("Value"=FALSE) -> ()  [unwired: 2 in, 2 out]
      n292 = property on="E" class="Bool (strict)"("Value"=FALSE) -> ()  [unwired: 2 in, 2 out]
      n293 = property on="D#" class="Bool (strict)"("Value"=FALSE) -> ()  [unwired: 2 in, 2 out]
      n294 = property on="D" class="Bool (strict)"("Value"=FALSE) -> ()  [unwired: 2 in, 2 out]
      n295 = property on="C#" class="Bool (strict)"("Value"=FALSE) -> ()  [unwired: 2 in, 2 out]
      n296 = property on="C" class="Bool (strict)"("Value"=FALSE) -> ()  [unwired: 2 in, 2 out]
      n297 = property on="D" class="Bool (strict)"("Value"=TRUE) -> ()  [unwired: 2 in, 2 out]
      n298 = property on="D#" class="Bool (strict)"("Value"=TRUE) -> ()  [unwired: 2 in, 2 out]
      n299 = property on="C#" class="Bool (strict)"("Value"=TRUE) -> ()  [unwired: 2 in, 2 out]
      n300 = property on="C" class="Bool (strict)"("Value"=TRUE) -> ()  [unwired: 2 in, 2 out]
      n301 = property on="G" class="Bool (strict)"("Value"=TRUE) -> ()  [unwired: 2 in, 2 out]
      n302 = property on="F" class="Bool (strict)"("Value"=TRUE) -> ()  [unwired: 2 in, 2 out]
      n303 = property on="F#" class="Bool (strict)"("Value"=TRUE) -> ()  [unwired: 2 in, 2 out]
      n304 = property on="E" class="Bool (strict)"("Value"=TRUE) -> ()  [unwired: 2 in, 2 out]
      n305 = property on="G#" class="Bool (strict)"("Value"=TRUE) -> ()  [unwired: 2 in, 2 out]
      n306 = property on="Bb" class="Bool (strict)"("Value"=TRUE) -> ()  [unwired: 2 in, 2 out]
      n307 = property on="B" class="Bool (strict)"("Value"=TRUE) -> ()  [unwired: 2 in, 2 out]
      n308 = property on="A" class="Bool (strict)"("Value"=TRUE) -> ()  [unwired: 2 in, 2 out]
    }
    frame Enabled {
    }
  }
  n309 = disable-structure shown="Enabled" {
    frame Disabled {
      n310 = property on="Wave type" class="Knob (strict)" props=["Value"]() -> ()  [unwired: 2 in, 3 out]
      n311 = property on="HI freq" class="Knob (strict)" props=["Value"]() -> ()  [unwired: 2 in, 3 out]
      n312 = property on="Octave ch1" class="Knob (strict)" props=["Value"]() -> ()  [unwired: 2 in, 3 out]
      n313 = property on="Blend" class="Knob (strict)" props=["Value"]() -> ()  [unwired: 2 in, 3 out]
      n314 = property on="Octave ch2" class="Knob (strict)" props=["Value"]() -> ()  [unwired: 2 in, 3 out]
      n315 = property on="Transpose" class="Knob (strict)" props=["Value"]() -> ()  [unwired: 2 in, 3 out]
      n316 = property on="Volume" class="Knob (strict)" props=["Value"]() -> ()  [unwired: 2 in, 3 out]
      n317 = property on="Attack" class="Knob (strict)" props=["Value"]() -> ()  [unwired: 2 in, 3 out]
      n318 = property on="Decay" class="Knob (strict)" props=["Value"]() -> ()  [unwired: 2 in, 3 out]
      n319 = property on="Distortion" class="Knob (strict)" props=["Value"]() -> ()  [unwired: 2 in, 3 out]
      n320 = property on="LOW freq" class="Knob (strict)" props=["Value"]() -> ()  [unwired: 2 in, 3 out]
      n321 = property on="Wave type 2" class="Knob (strict)" props=["Value"]() -> ()  [unwired: 2 in, 3 out]
    }
    frame Enabled {
    }
  }
